vi "SRLATCH.vi"(5 "Reset":bool, 11 "Set":bool) -> (3 "Output":bool)   [LabVIEW 2014]
doc: "When S is given an input of true, this VI will be set on; it will stay true as long as it is set. The VI resets when the R input turns on; it will then return false and wait for S to turn on again.\n\nIf both inputs are true, the Set is given priority and the input is set to true."
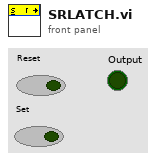
[diagram p1: front panel]
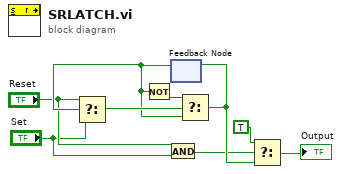
[diagram p0: block diagram]
diagram:
  n1 = And(x="Reset", y="Set") -> (x .and. y?=w4:bool)
  n2 = feedback #1() -> (w7:bool)  [unwired: 1 in]
  n3 = Select(t="Reset", s=w7, f="Set") -> (s? t:f=w9:bool)
  n4 = Not(x=w7) -> (.not. x?=w8:bool)
  n5 = Select(t=w8, s=w9, f=w7) -> (s? t:f=w5:bool)
  n6 = feedback-in #1(w5) -> ()
  n7 = Select(t=TRUE, s=w4, f=w5) -> (s? t:f=→"Output":bool)
